vi "buildDict.vi"(8 "error in (no error)":errorcluster, 11 "Map in":map{string, refnum<class "IBaseObject.lvclass">}(c390)) -> (0 "error out":errorcluster, 3 "IDict out":refnum<class "IDict.lvclass">)   [LabVIEW 2022 SP3, in "openDAQ.lvlib" / "daqUtils.lvlib"]
uses:
  daqUtils.lvlib
  daqCoreTypes/IDict/IDict.lvclass
  IBaseObject/IBaseObject.lvclass
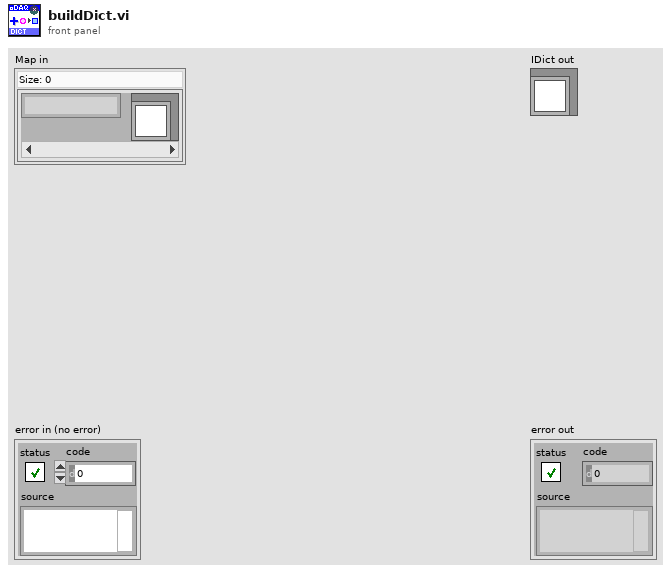
[diagram p1: front panel]
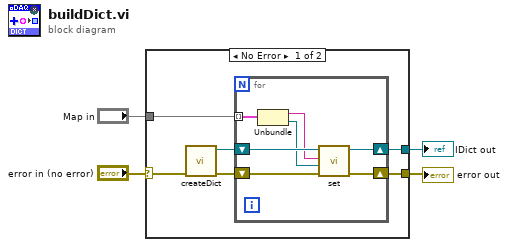
[diagram p0: block diagram]
diagram:
  n1 = case shown="No Error" "error in (no error)" {
    selector: "error in (no error)" -> [w10 w18]
    tunnel: [w6 w18] -> w4
    tunnel: "Map in" -> [w9 _]
    tunnel: [w5 _] -> w1
    frame No Error {
      n2 = call "createDict.vi"("error in (no error)"=w10) -> ("error out"=w7:errorcluster, "IDict out"=w8:refnum<class "IDict.lvclass">)  [unwired: 9 in]
      n3 = for {
        tunnel: w9 -> [w17] mode=indexing
        shift-right: [w15] -> w5
        shift-left: w8 -> [w16]
        shift-right: [w13] -> w6
        shift-left: w7 -> [w14]
        n4 = Unbundle(w17) -> (w12:string, "openDAQ.lvlib:IBaseObject.lvlib:IBaseObject.lvclass"=w11:refnum<class "IBaseObject.lvclass">)
        n5 = call "set.vi"("error in (no error)"=w14, "Value in"=w11, "Key in"=w12, "IDict in"=w16) -> ("error out"=w13:errorcluster, "IDict out"=w15:refnum<class "IDict.lvclass">)  [unwired: 5 in, 1 out]
      }
    }
    frame Error {
    }
  }
  "error out" <- w4
  "IDict out" <- w1
